vi "SearchAliasePXIDevice.vi"(8 "error in (no error)":errorcluster, 11 "SearchDevice":T2(ring)) -> (0 "error out":errorcluster, 3 "aliasDevice":string)   [LabVIEW 2017]
uses:
  <vilib>/nisyscfg/Expert Info.ctl
  <vilib>/nisyscfg/Close (Hardware).vi
  <vilib>/nisyscfg/Close (System).vi
  <vilib>/nisyscfg/nisyscfg.lvlib
  <resource>/objmgr/niMIDebugSession.rc
  <resource>/objmgr/nicontrollersysapi.rc
panel:
  out "Supported Experts":T1[](array[typedef])
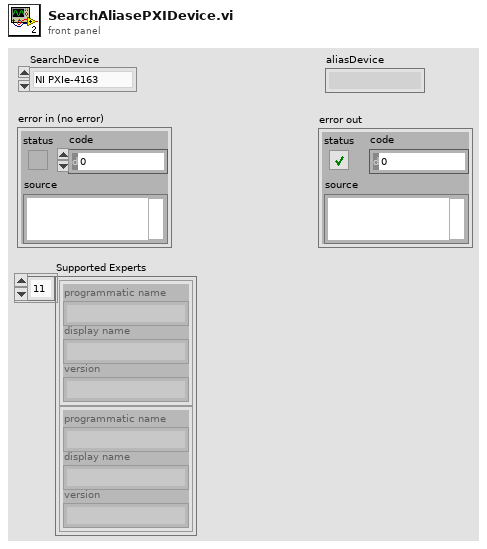
[diagram p1: front panel]
types:
  T1 = typedef "nisyscfg.lvlib/Expert Info.ctl" = cluster{"programmatic name":string, "display name":string, "version":string}
  T2 = enum16{"NI PXIe-4163", "NI PXIe-4135", "NI PXIe-4139", "NI PXIe-4112", "NI PXIe-4113", "NI PXIe-2532B", "NI PXIe-4081"}
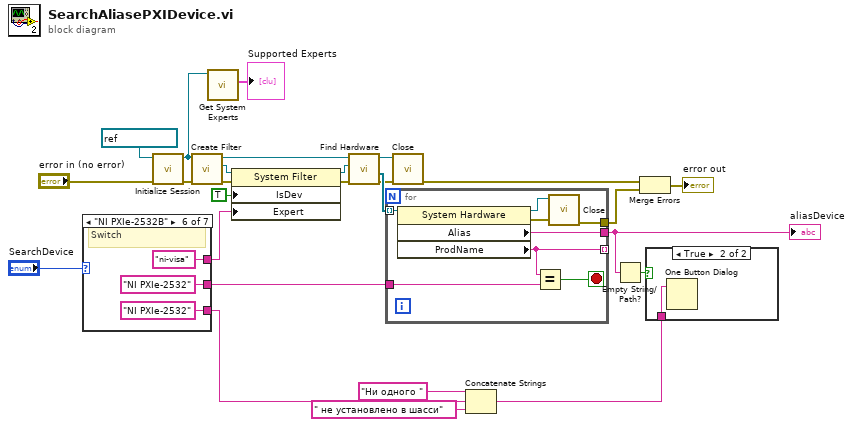
[diagram p0: block diagram]
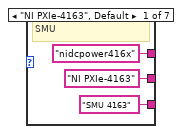
[diagram p2: hidden frame]
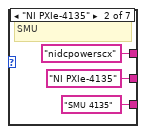
[diagram p3: hidden frame]
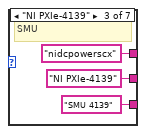
[diagram p4: hidden frame]
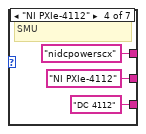
[diagram p5: hidden frame]
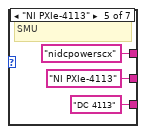
[diagram p6: hidden frame]
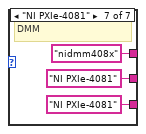
[diagram p7: hidden frame]
diagram:
  n1 = case shown="\"NI PXIe-2532B\"" "SearchDevice" {
    tunnel: ["nidcpower416x" ("Experts") "nidcpowerscx" ("Experts") "nidcpowerscx" ("Experts") "nidcpowerscx" ("Experts") "nidcpowerscx" ("Experts") "ni-visa" ("Experts") "nidmm408x" ("Experts")] -> w6
    tunnel: ["SMU 4163" ("Experts") "SMU 4135" ("Experts") "SMU 4139" ("Experts") "DC 4112" ("Experts") "DC 4113" ("Experts") "NI PXIe-2532" ("Experts") "NI PXIe-4081" ("Experts")] -> w7
    tunnel: ["NI PXIe-4163" ("searchDevice") "NI PXIe-4135" ("searchDevice") "NI PXIe-4139" ("searchDevice") "NI PXIe-4112" ("searchDevice") "NI PXIe-4113" ("searchDevice") "NI PXIe-2532" ("searchDevice") "NI PXIe-4081" ("searchDevice")] -> w8
    frame "NI PXIe-4163", Default {
      # "SMU"
    }
    frame "NI PXIe-4135" {
      # "SMU"
    }
    frame "NI PXIe-4139" {
      # "SMU"
    }
    frame "NI PXIe-4112" {
      # "SMU"
    }
    frame "NI PXIe-4113" {
      # "SMU"
    }
    frame "NI PXIe-2532B" {
      # "Switch"
    }
    frame "NI PXIe-4081" {
      # "DMM"
    }
  }
  n2 = call <vilib>:"Initialize Session.vi"("error in (no error)"="error in (no error)", "Target (localhost)"=refnum<k21> "localhost") -> ("error out"=w22:errorcluster, "Session out"=w2:refnum<k21>)  [unwired: 8 in]
  n3 = call <vilib>:"Create Filter.vi"("error in (no error)"=w22, "Session in"=w2) -> ("error out"=w19:errorcluster, "Filter out"=w20:refnum<k20>, "Session out"=w23:refnum<k21>)  [unwired: 7 in]
  n4 = call <vilib>:"Get System Experts.vi"("Session in"=w2) -> ("Supported Experts"=→"Supported Experts":T1[])  [unwired: 8 in, 2 out]
  n5 = property class="System Filter"(reference=w20, error in=w19, "IsDev"=TRUE ("Is Device"), "Expert"=w6) -> (reference out=w21:refnum<k20>, error out=w25:errorcluster)
  n6 = call <vilib>:"Find Hardware.vi"("error in (no error)"=w25, "Filter in"=w21, "Session in"=w23) -> ("error out"=w15:errorcluster, "Resources out"=w24:refnum<k20>[], "Session out"=w14:refnum<k21>)  [unwired: 5 in, 1 out]
  n7 = for {
    tunnel: w24 -> [w55] mode=indexing
    tunnel: [w49] -> w16
    tunnel: [w48] -> _ mode=indexing
    tunnel: w8 -> [w51]
    tunnel: [w50] -> w4
    stop <- w54 stop-if-true
    n8 = property class="System Hardware"(reference=w55) -> (reference out=w52:refnum<k20>, error out=w53:errorcluster, "Alias"=w49:string, "ProdName"=w48:string)  [unwired: 1 in]
    n9 = Equal?(x=w48, y=w51) -> (x = y?=w54:bool)
    n10 = call-poly <vilib>:"Close.vi"("error in (no error)"=w53, "Resource in"=w52) -> ("error out"=w50:errorcluster)  [unwired: 9 in]
  }
  "aliasDevice" <- w16
  n11 = call-poly <vilib>:"Close.vi"("error in (no error)"=w15, "Session in"=w14) -> ("error out"=w5:errorcluster)  [unwired: 9 in]
  n12 = Concatenate Strings("Ни одного ", w7, " не установлено в шасси" ("string")) -> (w10:string)
  n13 = Empty String/Path?(string/path=w16) -> (empty?=w26:bool)
  n14 = Merge Errors(w5, w4) -> (→"error out":errorcluster)
  n15 = case shown="True" w26 {
    tunnel: w10 -> [_ w56]
    frame False {
    }
    frame True {
      n16 = One Button Dialog(message=w56) -> ()  [unwired: 1 in, 1 out]
    }
  }
